vi "test change fails and produces message and actual file.vi"(8 "error in (no error)":errorcluster, 11 "TestCase in":refnum<class "Testing Approval Tests.lvclass">) -> (0 "error out":errorcluster, 3 "TestCase out":refnum<class "Testing Approval Tests.lvclass">)   [LabVIEW 2020, in "Testing Approval Tests.lvclass"]
uses:
  Testing Approval Tests.lvclass
  <vilib>/addons/_JKI Toolkits/VI Tester/TestCase.llb/TestCase.lvclass
  Approval Tests/Approval Tests.lvlib
  C:/Program Files/National Instruments/LabVIEW 2020/vi.lib/addons/_JKI Toolkits/VI Tester/TestCase.llb/TestCase.lvclass
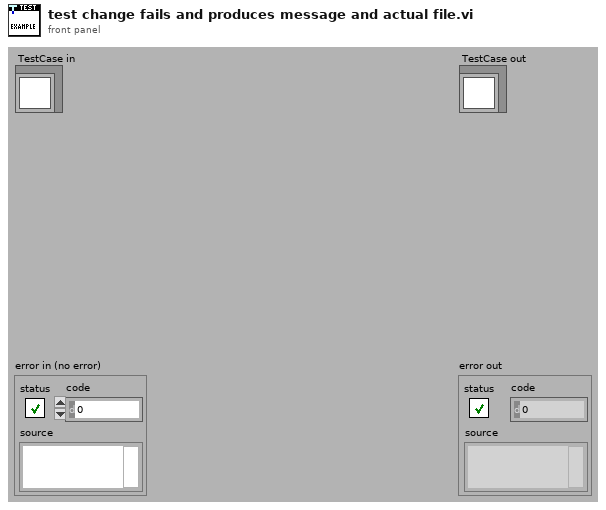
[diagram p1: front panel]
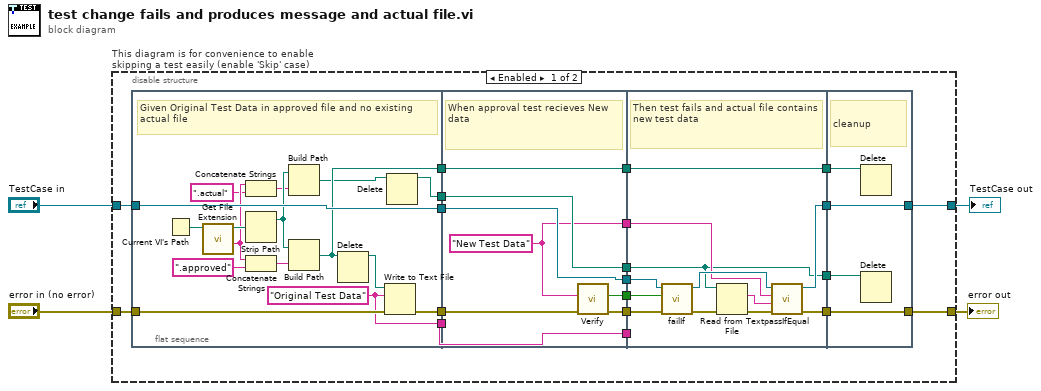
[diagram p0: block diagram]
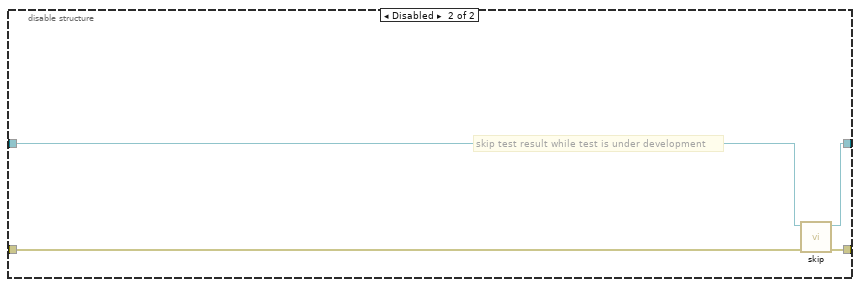
[diagram p2: hidden frame]
diagram:
  n1 = disable-structure "This diagram is for convenience to enable skipping a test easily (enable 'Skip' case)" shown="Enabled" {
    disable-tunnel: "TestCase in" -> [w16 w68]
    disable-tunnel: [w15 w66] -> w1
    disable-tunnel: [w23 w67] -> w3
    disable-tunnel: "error in (no error)" -> [w24 w65]
    frame Enabled {
      n2 = flat-sequence {
        tunnel: w24 -> [w36]
        tunnel: [w35] -> w22
        tunnel: [w40] -> w17
        tunnel: w16 -> [w40]
        tunnel: [w33] -> w11
        tunnel: [w26] -> w9
        tunnel: [w25] -> w7
        tunnel: w22 -> [w47]
        tunnel: [w46] -> w21
        tunnel: [w48] -> w18
        tunnel: w17 -> [w48]
        tunnel: [w42] -> w14
        tunnel: [w45] -> w12
        tunnel: w11 -> [w45]
        tunnel: [w44] -> w10
        tunnel: w9 -> [w44]
        tunnel: [w41] -> w8
        tunnel: w7 -> [w43]
        tunnel: [w43] -> w6
        tunnel: w21 -> [w60]
        tunnel: [w54] -> w20
        tunnel: [w52] -> w19
        tunnel: w18 -> [w58]
        tunnel: w14 -> [w57]
        tunnel: [w56] -> w13
        tunnel: w12 -> [w56]
        tunnel: w10 -> [w49]
        tunnel: w8 -> [w51]
        tunnel: w6 -> [_]
        tunnel: [w49] -> w5
        tunnel: [w64] -> w23
        tunnel: w20 -> [w64]
        tunnel: [w63] -> w15
        tunnel: w19 -> [w63]
        tunnel: w13 -> [w62]
        tunnel: w5 -> [w61]
        frame #0 {
          w25 = "Original Test Data"
          # "Given Original Test Data in approved file and no existing actual file"
          n3 = Current VI's Path() -> (path=w39:path)
          n4 = call <vilib>:"Get File Extension.vi"("file"=w39) -> ("filename without extension"=w31:string, "dup file"=w38:path)  [unwired: 6 in, 3 out]
          n5 = Concatenate Strings(w31, ".actual" ("string")) -> (w27:string)
          n6 = Strip Path(path=w38) -> (stripped path=w28:path)  [unwired: 1 out]
          n7 = Concatenate Strings(w31, ".approved" ("string")) -> (w32:string)
          n8 = Build Path(base path=w28, name or relative path=w27) -> (appended path=w29:path)
          n9 = Build Path(base path=w28, name or relative path=w32) -> (appended path=w33:path)
          n10 = Delete(path (use dialog)=w33) -> (deleted path=w34:path)  [unwired: 4 in, 2 out]
          n11 = Write to Text File(file (use dialog)=w34, text=w25, error in=w36) -> (error out=w35:errorcluster)  [unwired: 1 in, 2 out]
          n12 = Delete(path (use dialog)=w29) -> (deleted path=w26:path)  [unwired: 4 in, 2 out]
        }
        frame #1 {
          w41 = "New Test Data"
          # "When approval test recieves New data"
          n13 = call "Verify.vi"("error in"=w47, "Test Data"=w41) -> ("error out"=w46:errorcluster, "Passed?"=w42:bool)  [unwired: 7 in, 1 out]
        }
        frame #2 {
          # "Then test fails and actual file contains new test data"
          n14 = call-dynamic "failIf.vi"("error in (no error)"=w60, "fail"=w57, "TestCase in"=w58) -> ("error out"=w59:errorcluster, "TestCase out"=w53:refnum<class "Testing Approval Tests.lvclass">)  [unwired: 7 in]
          n15 = Read from Text File(file (use dialog)=w49, error in=w59) -> (text=w50:string, error out=w55:errorcluster)  [unwired: 2 in, 2 out]
          n16 = call-dynamic "passIfEqual.vi"("error in (no error)"=w55, "y"=w50, "x"=w51, "TestCase in"=w53) -> ("error out"=w54:errorcluster, "TestCase out"=w52:refnum<class "Testing Approval Tests.lvclass">)  [unwired: 6 in]
        }
        frame #3 {
          # "cleanup"
          n17 = Delete(path (use dialog)=w62) -> ()  [unwired: 4 in, 3 out]
          n18 = Delete(path (use dialog)=w61) -> ()  [unwired: 4 in, 3 out]
        }
      }
    }
    frame Disabled {
      # "skip test result while test is under development"
      n19 = call <vilib>:"skip.vi"("error in (no error)"=w65, "TestCase in"=w68) -> ("error out"=w67:errorcluster, "TestCase out"=w66:refnum<class "Testing Approval Tests.lvclass">)  [unwired: 8 in]
    }
  }
  "error out" <- w3
  "TestCase out" <- w1
